vi "Compute State Sequence.vi"(0 "Parent Action":T2, 2 "Buttons (in)":T1, 3 "error in (no error)":errorcluster) -> (6 "Action Sequence":cluster{"LCOS State":T3, "Data":variant}[](array[cluster]), 7 "Buttons (out)":T1, 9 "error out":errorcluster)   [LabVIEW 2011]
uses:
  LCOS State Machine States.ctl
  LCOS Parent Action.ctl
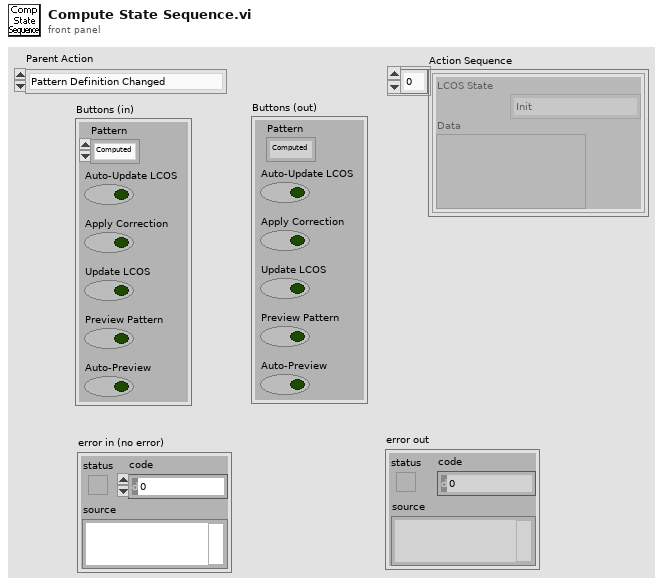
[diagram p1: front panel]
types:
  T1 = cluster{"Pattern":enum16{"Computed", "From File", "Correction"}, "Auto-Update LCOS":bool, "Apply Correction":bool, "Update LCOS":bool, "Preview Pattern":bool, "Auto-Preview":bool}
  T2 = typedef "LCOS Parent Action.ctl" = enum16{"Pattern Definition Changed", "Preview Button Pushed", "Update Button Pushed", "Pattern Selection Changed", "Correction Pattern Changed", "User Pattern (from File) Changed"}
  T3 = typedef "LCOS State Machine States.ctl" = enum16{"Init", "Idle", "Preview Button Pushed", "Update Button Pushed", "Pattern Selection Changed", "Pattern Definition Changed", "Selected File Changed", "Load Correction Pattern", "Load Correction Pattern Step 2", "Load User Pattern", "Load User Pattern Step 2", "Compute Pattern", "Correct Pattern", "Update Preview Display", "Update LCOS Display", "Error", "Clear Error", "Exit"}
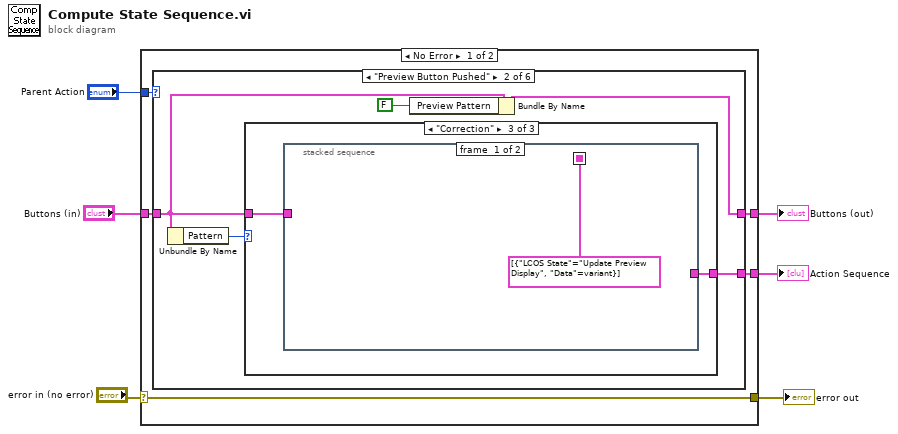
[diagram p0: block diagram]
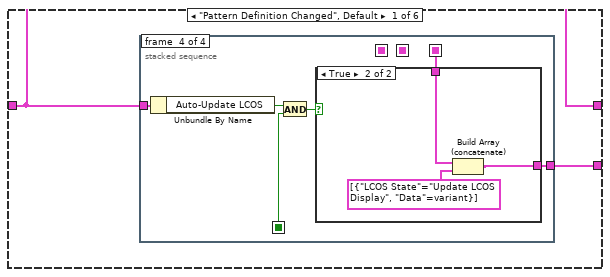
[diagram p2: hidden frame]
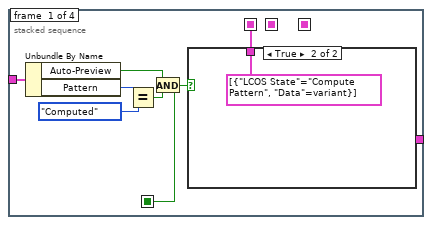
[diagram p3: hidden frame]
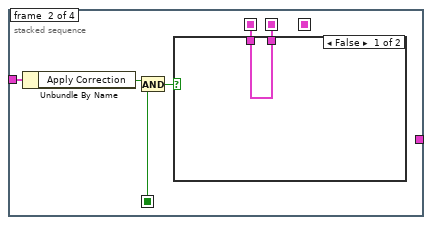
[diagram p5: hidden frame]
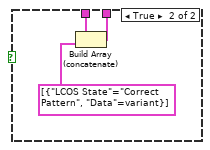
[diagram p6: hidden frame]
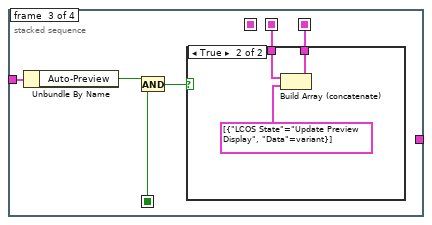
[diagram p7: hidden frame]
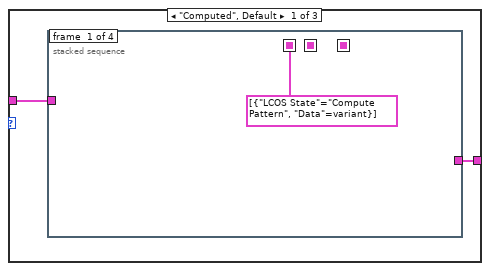
[diagram p10: hidden frame]
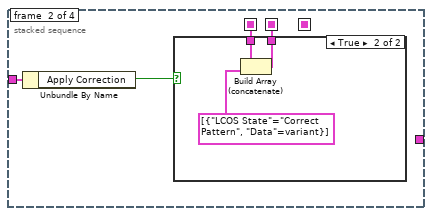
[diagram p11: hidden frame]
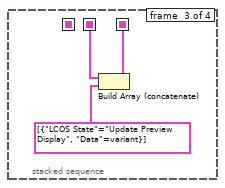
[diagram p13: hidden frame]
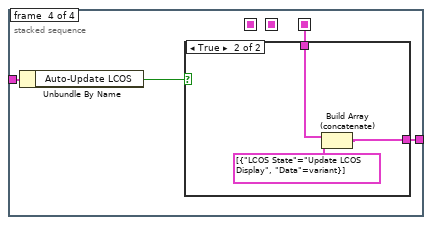
[diagram p14: hidden frame]
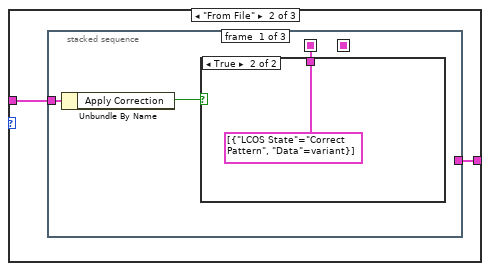
[diagram p16: hidden frame]
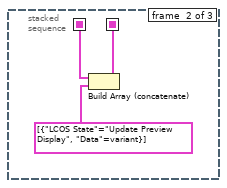
[diagram p18: hidden frame]
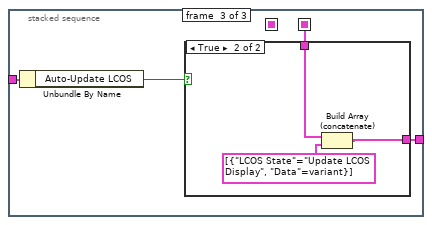
[diagram p19: hidden frame]
diagram:
  n1 = case shown="No Error" "error in (no error)" {
    selector: "error in (no error)" -> [w9 w186]
    tunnel: [w9 w186] -> w5
    tunnel: "Parent Action" -> [w11 _]
    tunnel: "Buttons (in)" -> [w10 w185]
    tunnel: [w8 w185] -> w2
    tunnel: [w7 _] -> w1
    frame No Error {
      n2 = case shown="\"Preview Button Pushed\"" w11 {
        tunnel: w10 -> [w13 w55 w110 w113 w183 w184]
        tunnel: [w13 w54 w108 w113 w183 w184] -> w8
        tunnel: [w12 w56 cluster{"LCOS State":T3, "Data":variant}[] [{"LCOS State"=enum."Update LCOS Display", "Data"=variant}] ("Action Sequence") w111 _ _] -> w7
        frame "Pattern Definition Changed", Default {
          n3 = stacked-sequence {
            seq-local: [w15 _ _ _] -> [_ w25 _ _]
            seq-local: [w14 _ _ _] -> [_ w23 w35 w45]
            seq-local: [_ w24 _ _] -> [_ _ w33 _]
            seq-local: [_ _ w32 _] -> [_ _ _ w43]
            tunnel: w13 -> [w20 w27 w37 w47]
            tunnel: [_ _ _ w42] -> w12
            frame #0 {
              n4 = Unbundle By Name(w20) -> ("Auto-Preview"=w17:bool, "Pattern"=w19:enum16{"Computed", "From File", "Correction"})
              n5 = Equal?(x=w19, y=enum16{"Computed", "From File", "Correction"}."Computed" ("Pattern")) -> (x = y?=w16:bool)
              n6 = And(x=w17, y=w16) -> (x .and. y?=w14:bool)
              n7 = case shown="True" w14 {
                tunnel: [_ cluster{"LCOS State":T3, "Data":variant}[] [{"LCOS State"=enum."Compute Pattern", "Data"=variant}] ("Action Sequence")] -> w15
                frame False {
                }
                frame True {
                }
              }
            }
            frame #1 {
              n8 = Unbundle By Name(w27) -> ("Apply Correction"=w22:bool)
              n9 = And(x=w22, y=w23) -> (x .and. y?=w26:bool)
              n10 = case shown="False" w26 {
                tunnel: w25 -> [w28 w31]
                tunnel: [w28 w29] -> w24
                frame False {
                }
                frame True {
                  n11 = Build Array (concatenate)(w31, cluster{"LCOS State":T3, "Data":variant}[] [{"LCOS State"=enum."Correct Pattern", "Data"=variant}] ("Action Sequence")) -> (w29:cluster{"LCOS State":T3, "Data":variant}[])
                }
              }
            }
            frame #2 {
              n12 = Unbundle By Name(w37) -> ("Auto-Preview"=w36:bool)
              n13 = And(x=w36, y=w35) -> (x .and. y?=w34:bool)
              n14 = case shown="True" w34 {
                tunnel: w33 -> [w38 w41]
                tunnel: [w38 w39] -> w32
                frame False {
                }
                frame True {
                  n15 = Build Array (concatenate)(w41, cluster{"LCOS State":T3, "Data":variant}[] [{"LCOS State"=enum."Update Preview Display", "Data"=variant}] ("Action Sequence")) -> (w39:cluster{"LCOS State":T3, "Data":variant}[])
                }
              }
            }
            frame #3 {
              n16 = Unbundle By Name(w47) -> ("Auto-Update LCOS"=w46:bool)
              n17 = And(x=w46, y=w45) -> (x .and. y?=w44:bool)
              n18 = case shown="True" w44 {
                tunnel: w43 -> [w48 w51]
                tunnel: [w48 w49] -> w42
                frame False {
                }
                frame True {
                  n19 = Build Array (concatenate)(w51, cluster{"LCOS State":T3, "Data":variant}[] [{"LCOS State"=enum."Update LCOS Display", "Data"=variant}] ("Action Sequence")) -> (w49:cluster{"LCOS State":T3, "Data":variant}[])
                }
              }
            }
          }
        }
        frame "Preview Button Pushed" {
          n20 = Unbundle By Name(w55) -> ("Pattern"=w52:enum16{"Computed", "From File", "Correction"})
          n21 = case shown="\"Correction\"" w52 {
            tunnel: [w58 w80 w97] -> w56
            tunnel: w55 -> [w57 w79 w96]
            frame "Computed", Default {
              n22 = stacked-sequence {
                seq-local: [cluster{"LCOS State":T3, "Data":variant}[] [{"LCOS State"=enum."Compute Pattern", "Data"=variant}] ("Action Sequence") _ _ _] -> [_ w62 _ _]
                seq-local: [_ w61 _ _] -> [_ _ w70 _]
                seq-local: [_ _ w69 _] -> [_ _ _ w73]
                tunnel: w57 -> [_ w63 _ w74]
                tunnel: [_ _ _ w72] -> w58
                frame #0 {
                }
                frame #1 {
                  n23 = Unbundle By Name(w63) -> ("Apply Correction"=w60:bool)
                  n24 = case shown="True" w60 {
                    tunnel: w62 -> [w64 w67]
                    tunnel: [w64 w65] -> w61
                    frame False {
                    }
                    frame True {
                      n25 = Build Array (concatenate)(w67, cluster{"LCOS State":T3, "Data":variant}[] [{"LCOS State"=enum."Correct Pattern", "Data"=variant}] ("Action Sequence")) -> (w65:cluster{"LCOS State":T3, "Data":variant}[])
                    }
                  }
                }
                frame #2 {
                  n26 = Build Array (concatenate)(w70, cluster{"LCOS State":T3, "Data":variant}[] [{"LCOS State"=enum."Update Preview Display", "Data"=variant}] ("Action Sequence")) -> (w69:cluster{"LCOS State":T3, "Data":variant}[])
                }
                frame #3 {
                  n27 = Unbundle By Name(w74) -> ("Auto-Update LCOS"=w71:bool)
                  n28 = case shown="True" w71 {
                    tunnel: w73 -> [w75 w78]
                    tunnel: [w75 w76] -> w72
                    frame False {
                    }
                    frame True {
                      n29 = Build Array (concatenate)(w78, cluster{"LCOS State":T3, "Data":variant}[] [{"LCOS State"=enum."Update LCOS Display", "Data"=variant}] ("Action Sequence")) -> (w76:cluster{"LCOS State":T3, "Data":variant}[])
                    }
                  }
                }
              }
            }
            frame "From File" {
              n30 = stacked-sequence {
                seq-local: [w82 _ _] -> [_ w87 _]
                seq-local: [_ w86 _] -> [_ _ w90]
                tunnel: w79 -> [w83 _ w91]
                tunnel: [_ _ w89] -> w80
                frame #0 {
                  n31 = Unbundle By Name(w83) -> ("Apply Correction"=w81:bool)
                  n32 = case shown="True" w81 {
                    tunnel: [_ cluster{"LCOS State":T3, "Data":variant}[] [{"LCOS State"=enum."Correct Pattern", "Data"=variant}] ("Action Sequence")] -> w82
                    frame False {
                    }
                    frame True {
                    }
                  }
                }
                frame #1 {
                  n33 = Build Array (concatenate)(w87, cluster{"LCOS State":T3, "Data":variant}[] [{"LCOS State"=enum."Update Preview Display", "Data"=variant}] ("Action Sequence")) -> (w86:cluster{"LCOS State":T3, "Data":variant}[])
                }
                frame #2 {
                  n34 = Unbundle By Name(w91) -> ("Auto-Update LCOS"=w88:bool)
                  n35 = case shown="True" w88 {
                    tunnel: w90 -> [w92 w95]
                    tunnel: [w92 w93] -> w89
                    frame False {
                    }
                    frame True {
                      n36 = Build Array (concatenate)(w95, cluster{"LCOS State":T3, "Data":variant}[] [{"LCOS State"=enum."Update LCOS Display", "Data"=variant}] ("Action Sequence")) -> (w93:cluster{"LCOS State":T3, "Data":variant}[])
                    }
                  }
                }
              }
            }
            frame "Correction" {
              n37 = stacked-sequence {
                seq-local: [cluster{"LCOS State":T3, "Data":variant}[] [{"LCOS State"=enum."Update Preview Display", "Data"=variant}] ("Action Sequence") _] -> [_ w101]
                tunnel: w96 -> [_ w102]
                tunnel: [_ w100] -> w97
                frame #0 {
                }
                frame #1 {
                  n38 = Unbundle By Name(w102) -> ("Auto-Update LCOS"=w99:bool)
                  n39 = case shown="True" w99 {
                    tunnel: w101 -> [w103 w106]
                    tunnel: [w103 w104] -> w100
                    frame False {
                    }
                    frame True {
                      n40 = Build Array (concatenate)(w106, cluster{"LCOS State":T3, "Data":variant}[] [{"LCOS State"=enum."Update LCOS Display", "Data"=variant}] ("Action Sequence")) -> (w104:cluster{"LCOS State":T3, "Data":variant}[])
                    }
                  }
                }
              }
            }
          }
          n41 = Bundle By Name(cluster=w55, "Preview Pattern"=FALSE) -> (w54:T1)
        }
        frame "Update Button Pushed" {
          n42 = Bundle By Name(cluster=w110, "Update LCOS"=FALSE) -> (w108:T1)
        }
        frame "Pattern Selection Changed" {
          n43 = Unbundle By Name(w113) -> ("Pattern"=w112:enum16{"Computed", "From File", "Correction"})
          n44 = case shown="\"Correction\"" w112 {
            tunnel: [w115 w144 w168] -> w111
            tunnel: w113 -> [w114 w143 w167]
            frame "Computed", Default {
              n45 = stacked-sequence {
                seq-local: [cluster{"LCOS State":T3, "Data":variant}[] [{"LCOS State"=enum."Compute Pattern", "Data"=variant}] ("Action Sequence") _ _ _] -> [_ w119 _ _]
                seq-local: [_ w118 _ _] -> [_ _ w128 _]
                seq-local: [_ _ w127 _] -> [_ _ _ w137]
                seq-local: [_ _ w125 _] -> [_ _ _ w134]
                tunnel: w114 -> [_ w120 w126 w138]
                tunnel: [_ _ _ w136] -> w115
                frame #0 {
                }
                frame #1 {
                  n46 = Unbundle By Name(w120) -> ("Apply Correction"=w117:bool)
                  n47 = case shown="True" w117 {
                    tunnel: w119 -> [w121 w124]
                    tunnel: [w121 w122] -> w118
                    frame False {
                    }
                    frame True {
                      n48 = Build Array (concatenate)(w124, cluster{"LCOS State":T3, "Data":variant}[] [{"LCOS State"=enum."Correct Pattern", "Data"=variant}] ("Action Sequence")) -> (w122:cluster{"LCOS State":T3, "Data":variant}[])
                    }
                  }
                }
                frame #2 {
                  n49 = Unbundle By Name(w126) -> ("Auto-Preview"=w125:bool)
                  n50 = case shown="True" w125 {
                    tunnel: w128 -> [w129 w132]
                    tunnel: [w129 w130] -> w127
                    frame False {
                    }
                    frame True {
                      n51 = Build Array (concatenate)(w132, cluster{"LCOS State":T3, "Data":variant}[] [{"LCOS State"=enum."Update Preview Display", "Data"=variant}] ("Action Sequence")) -> (w130:cluster{"LCOS State":T3, "Data":variant}[])
                    }
                  }
                }
                frame #3 {
                  n52 = Unbundle By Name(w138) -> ("Auto-Update LCOS"=w135:bool)
                  n53 = And(x=w134, y=w135) -> (x .and. y?=w133:bool)
                  n54 = case shown="True" w133 {
                    tunnel: w137 -> [w139 w142]
                    tunnel: [w139 w140] -> w136
                    frame False {
                    }
                    frame True {
                      n55 = Build Array (concatenate)(w142, cluster{"LCOS State":T3, "Data":variant}[] [{"LCOS State"=enum."Update LCOS Display", "Data"=variant}] ("Action Sequence")) -> (w140:cluster{"LCOS State":T3, "Data":variant}[])
                    }
                  }
                }
              }
            }
            frame "From File" {
              n56 = stacked-sequence {
                seq-local: [w146 _ _] -> [_ w152 _]
                seq-local: [_ w151 _] -> [_ _ w161]
                seq-local: [_ w149 _] -> [_ _ w158]
                tunnel: w143 -> [w147 w150 w162]
                tunnel: [_ _ w160] -> w144
                frame #0 {
                  n57 = Unbundle By Name(w147) -> ("Apply Correction"=w145:bool)
                  n58 = case shown="True" w145 {
                    tunnel: [_ cluster{"LCOS State":T3, "Data":variant}[] [{"LCOS State"=enum."Correct Pattern", "Data"=variant}] ("Action Sequence")] -> w146
                    frame False {
                    }
                    frame True {
                    }
                  }
                }
                frame #1 {
                  n59 = Unbundle By Name(w150) -> ("Auto-Preview"=w149:bool)
                  n60 = case shown="False" w149 {
                    tunnel: w152 -> [w153 w156]
                    tunnel: [w153 w155] -> w151
                    frame False {
                    }
                    frame True {
                      n61 = Build Array (concatenate)(w156, cluster{"LCOS State":T3, "Data":variant}[] [{"LCOS State"=enum."Update Preview Display", "Data"=variant}] ("Action Sequence")) -> (w155:cluster{"LCOS State":T3, "Data":variant}[])
                    }
                  }
                }
                frame #2 {
                  n62 = Unbundle By Name(w162) -> ("Auto-Update LCOS"=w159:bool)
                  n63 = And(x=w158, y=w159) -> (x .and. y?=w157:bool)
                  n64 = case shown="True" w157 {
                    tunnel: w161 -> [w163 w166]
                    tunnel: [w163 w164] -> w160
                    frame False {
                    }
                    frame True {
                      n65 = Build Array (concatenate)(w166, cluster{"LCOS State":T3, "Data":variant}[] [{"LCOS State"=enum."Update LCOS Display", "Data"=variant}] ("Action Sequence")) -> (w164:cluster{"LCOS State":T3, "Data":variant}[])
                    }
                  }
                }
              }
            }
            frame "Correction" {
              n66 = stacked-sequence {
                seq-local: [w171 _] -> [_ w177]
                seq-local: [w169 _] -> [_ w174]
                tunnel: w167 -> [w170 w178]
                tunnel: [_ w176] -> w168
                frame #0 {
                  n67 = Unbundle By Name(w170) -> ("Auto-Preview"=w169:bool)
                  n68 = case shown="True" w169 {
                    tunnel: [_ cluster{"LCOS State":T3, "Data":variant}[] [{"LCOS State"=enum."Update Preview Display", "Data"=variant}] ("Action Sequence")] -> w171
                    frame False {
                    }
                    frame True {
                    }
                  }
                }
                frame #1 {
                  n69 = Unbundle By Name(w178) -> ("Auto-Update LCOS"=w175:bool)
                  n70 = And(x=w174, y=w175) -> (x .and. y?=w173:bool)
                  n71 = case shown="True" w173 {
                    tunnel: w177 -> [w179 w182]
                    tunnel: [w179 w180] -> w176
                    frame False {
                    }
                    frame True {
                      n72 = Build Array (concatenate)(w182, cluster{"LCOS State":T3, "Data":variant}[] [{"LCOS State"=enum."Update LCOS Display", "Data"=variant}] ("Action Sequence")) -> (w180:cluster{"LCOS State":T3, "Data":variant}[])
                    }
                  }
                }
              }
            }
          }
        }
        frame "Correction Pattern Changed" {
        }
        frame "User Pattern (from File) Changed" {
        }
      }
    }
    frame Error {
    }
  }
  "Action Sequence" <- w1
  "error out" <- w5
  "Buttons (out)" <- w2
